vi "Load Rich Text Notebook.vi"(6 "Backup?":bool, 8 "Error In":errorcluster, 10 "File Path Control":path, 11 ".NET Refnum in":refnum<k24>) -> (0 "Error Out":errorcluster, 1 "cancelled":bool, 2 "File Path out":path, 3 ".NET Refnum out":refnum<k24>, 4 "RTF content":string)   [LabVIEW 2019, in "Notebook.lvlib"]
uses:
  Notebook.lvlib
  System.Windows.Forms
  Notebook Saved Global.vi
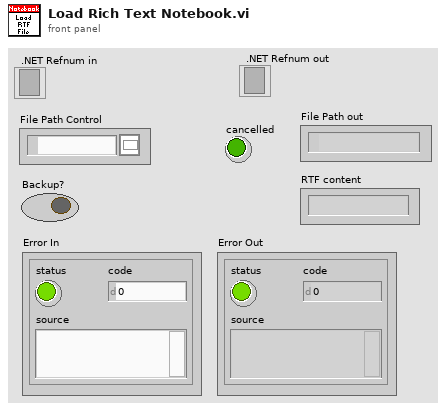
[diagram p1: front panel]
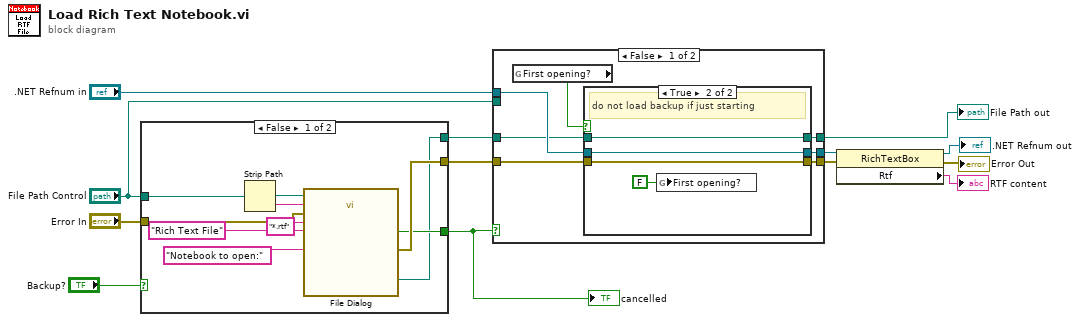
[diagram p0: block diagram]
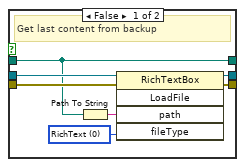
[diagram p3: hidden frame]
diagram:
  n1 = case shown="False" "Backup?" {
    tunnel: [w23 w24] -> w12
    tunnel: "Error In" -> [w22 w24]
    tunnel: [w16 _] -> w10
    tunnel: [w15 w25] -> w9
    tunnel: "File Path Control" -> [w14 w25]
    frame False {
      n2 = Strip Path(path=w14) -> (stripped path=w20:path, name=w19:string)
      n3 = call "File Dialog"("start path"=w20, "prompt"="Notebook to open:", "default name"=w19, "error in"=w22, "pattern (all files)"="*.rtf" ("pattern label"), "pattern label"="Rich Text File") -> ("selected path"=w15:path, "cancelled"=w16:bool, "error out"=w23:errorcluster)  [unwired: 6 in, 1 out]
    }
    frame True {
    }
  }
  "cancelled" <- w10
  n4 = case shown="False" w10 {
    tunnel: ".NET Refnum in" -> [w32 w44]
    tunnel: w12 -> [w31 w46]
    tunnel: [w29 w46] -> w6
    tunnel: w9 -> [w28 _]
    tunnel: [w26 w45] -> w8
    tunnel: "File Path Control" -> [_ w45]
    tunnel: [w30 w44] -> w7
    frame False {
      n5 = global read "Notebook Saved Global.vi" "First opening?"() -> (w27:bool)
      n6 = case shown="True" w27 {
        tunnel: w32 -> [w39 w41]
        tunnel: w31 -> [w38 w42]
        tunnel: [w36 w41] -> w30
        tunnel: [w35 w42] -> w29
        tunnel: w28 -> [w33 w40]
        tunnel: [w33 w40] -> w26
        frame False {
          w37 = 0 items=["RichText", "PlainText", "RichNoOleObjs", "TextTextOleObjs", "UnicodePlainText"] ("fileType")
          # "Get last content from backup"
          n7 = Path To String(path=w33) -> (string=w34:string)
          n8 = invoke class="RichTextBox" method="LoadFile"(reference=w39, error in=w38, "path"=w34, "fileType"=w37) -> (reference out=w36:refnum<k24>, error out=w35:errorcluster)  [unwired: 1 in, 3 out]
        }
        frame True {
          # "do not load backup if just starting"
          n9 = global write "Notebook Saved Global.vi" "First opening?"(FALSE ("First opening?")) -> ()
        }
      }
    }
    frame True {
    }
  }
  "File Path out" <- w8
  n10 = property class="RichTextBox"(reference=w7, error in=w6) -> (reference out=→".NET Refnum out":refnum<k24>, error out=→"Error Out":errorcluster, "Rtf"=→"RTF content":string)
